vi "Module_IniFile.vi"(7 "処理":enum16{"Read", "Get", "GetArray"}(ring), 8 "error in (no error)":errorcluster caption="エラー入力 (エラーなし)", 9 "一括取得キー":string[](array[string]), 10 "取得キー":string, 11 "ファイルパス":path=path "C:/Users/0128712/Documents/ヘルプファイル/LabVIEW/SampleVI/設定ファイル/ResolverAdj.dat") -> (0 "error out":errorcluster caption="エラー出力", 1 "一括取得データ":string[](array[string]), 3 "取得データ":string)   [LabVIEW 2018]
uses:
  <vilib>/Utility/config.llb/Read Key (String).vi
  <vilib>/Utility/config.llb/NI_LVConfig.lvlib
panel:
  out "読出値":T1(array[cluster])
  # "<機能>\n■Read\n　設定ファイルを読み込む\n　テキスト形式で有れば拡張子は問わない\n■Get\n　キーから値を取得する\n■GetArray\n　キーの配列からまとめて値を取得する\n　Getを複数まとめて行う"
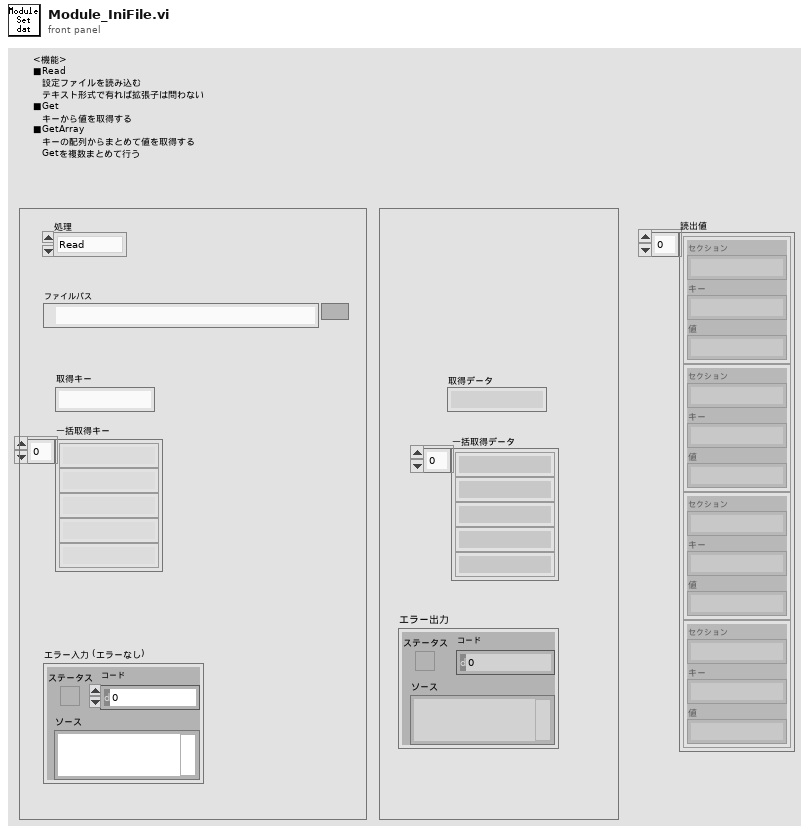
[diagram p1: front panel]
types:
  T1 = cluster{"セクション":string, "キー":string, "値":string}[]
  T2 = typedef "NI_LVConfig.lvlib/Config Data RefNum.ctl" = refnum<k1>
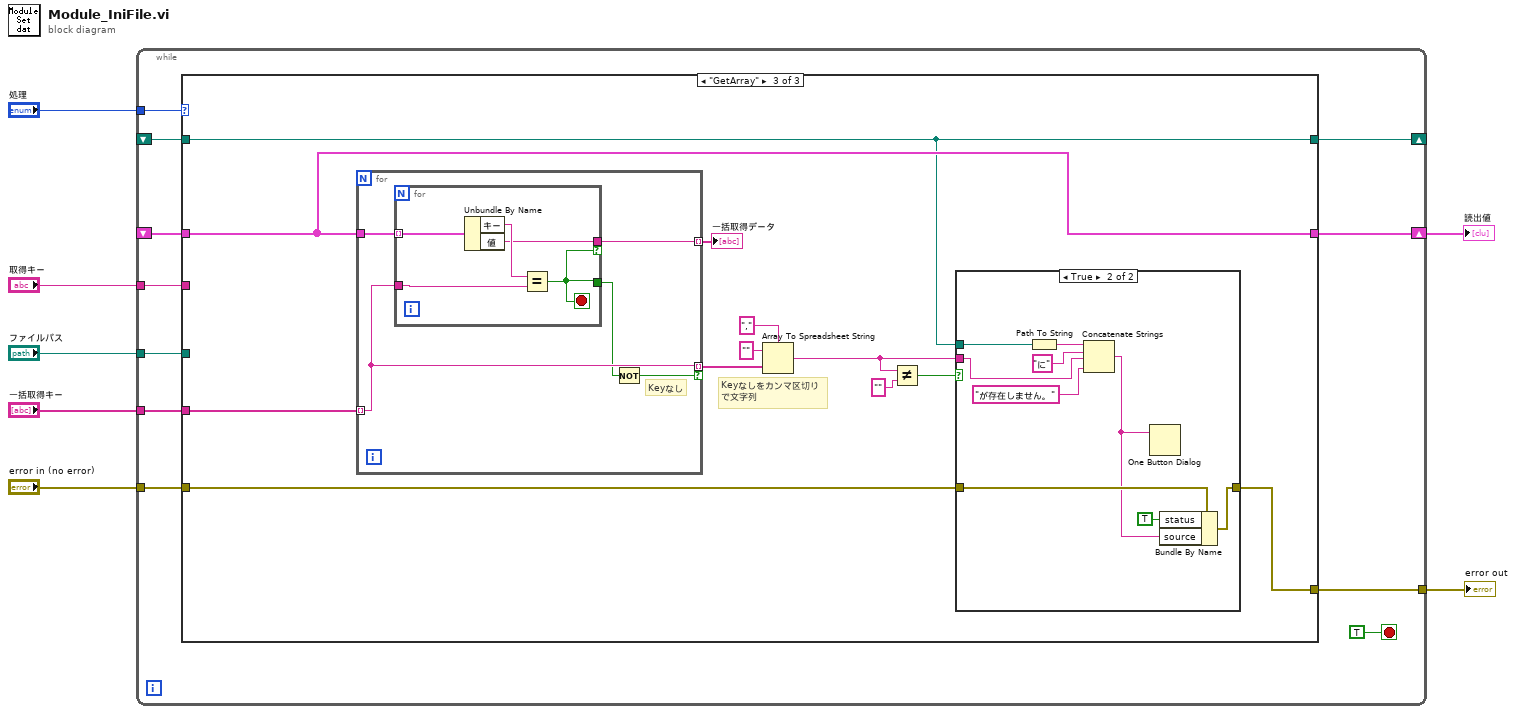
[diagram p0: block diagram]
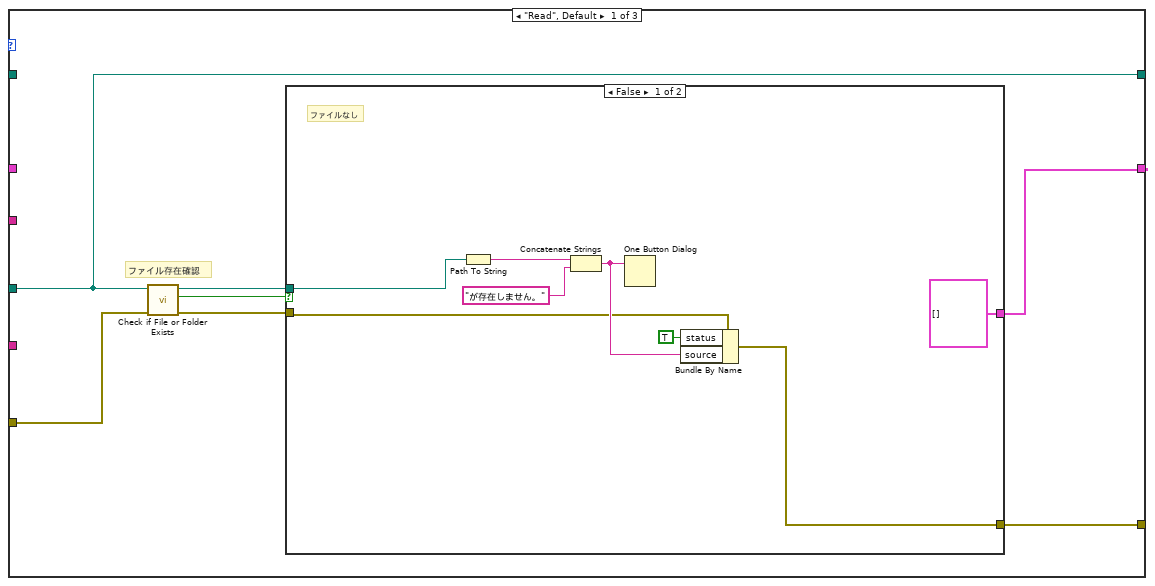
[diagram p2: hidden frame]
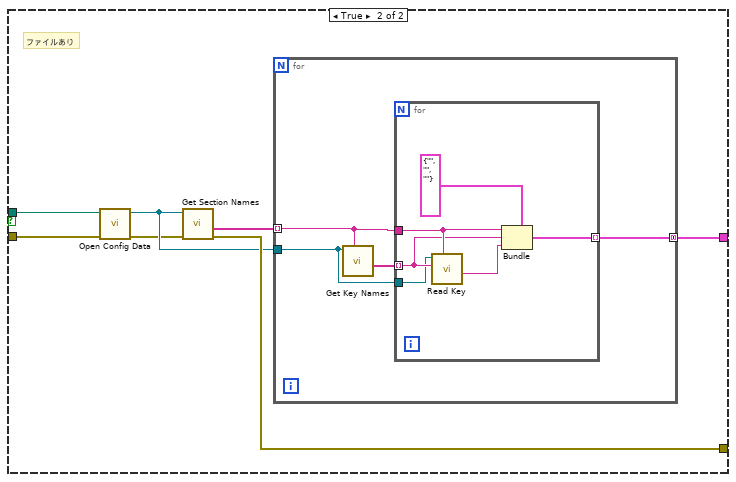
[diagram p3: hidden frame]
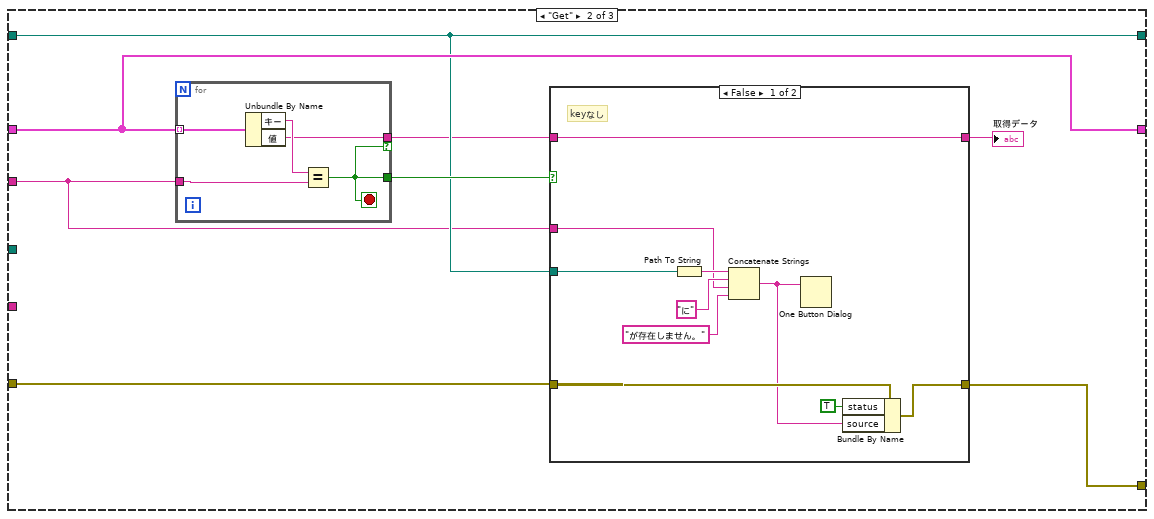
[diagram p4: hidden frame]
diagram:
  n1 = while {
    tunnel: "処理" -> [w17]
    tunnel: "ファイルパス" -> [w16]
    shift-right: [w15] -> w1
    shift-left: _ -> [w14]
    tunnel: "取得キー" -> [w13]
    tunnel: "error in (no error)" -> [w12]
    tunnel: [w11] -> w3
    tunnel: "一括取得キー" -> [w10]
    shift-right: [w9] -> _
    shift-left: _ -> [w8]
    stop <- TRUE stop-if-true
    n2 = case shown="\"GetArray\"" w17 {
      tunnel: w16 -> [w19 _ _]
      tunnel: [w24 w58 w87] -> w15
      tunnel: w14 -> [_ w58 w87]
      tunnel: w13 -> [_ w52 _]
      tunnel: w12 -> [w23 w55 w83]
      tunnel: [w25 w54 w82] -> w11
      tunnel: w10 -> [_ _ w86]
      tunnel: [w19 w53 w84] -> w9
      tunnel: w8 -> [_ w53 w84]
      frame "Read", Default {
        # "ファイル存在確認"
        n3 = call <vilib>:"Check if File or Folder Exists.vi"("error in (no error)"=w23, "path"=w19) -> ("error out"=w22:errorcluster, "file or folder exists?"=w20:bool, "dup path"=w21:path)  [unwired: 7 in]
        n4 = case shown="FALSE" w20 {
          tunnel: [w28 w40] -> w25
          tunnel: [T1 [] w36] -> w24
          tunnel: w22 -> [w29 w35]
          tunnel: w21 -> [w26 w34]
          frame False {
            # "ファイルなし"
            n5 = Path To String(path=w26) -> (string=w33:string)
            n6 = Concatenate Strings(w33, "が存在しません。") -> (w30:string)
            n7 = One Button Dialog(message=w30) -> ()  [unwired: 1 in, 1 out]
            n8 = Bundle By Name(cluster=w29, "status"=TRUE, "source"=w30) -> (w28:errorcluster)
          }
          frame True {
            # "ファイルあり"
            n9 = call <vilib>:"Open Config Data.vi"("error in (no error)"=w35, "configuration file path"=w34) -> ("error out"=w37:errorcluster, "refnum"=w38:T2)  [unwired: 7 in, 1 out]
            n10 = call <vilib>:"Get Section Names.vi"("error in (no error)"=w37, "refnum"=w38) -> ("error out"=w40:errorcluster, "section names"=w39:string[])  [unwired: 7 in, 1 out]
            n11 = for {
              tunnel: w39 -> [w43] mode=indexing
              tunnel: w38 -> [w42]
              tunnel: [w41] -> w36 mode=concatenating
              n12 = call <vilib>:"Get Key Names.vi"("section"=w43, "refnum"=w42) -> ("key names"=w44:string[])  [unwired: 6 in, 3 out]
              n13 = for {
                tunnel: w44 -> [w49] mode=indexing
                tunnel: w43 -> [w50]
                tunnel: w42 -> [w47]
                tunnel: [w46] -> w41 mode=indexing
                n14 = call-poly <vilib>:"Read Key.vi"("section"=w50, "key"=w49, "refnum"=w47) -> ("value"=w48:string)  [unwired: 5 in, 3 out]
                n15 = Bundle(cluster=cluster{"セクション":string, "キー":string, "値":string} {"セクション"="", "キー"="", "値"=""} ("クラスタ 2"), "セクション"=w50, "キー"=w49, "値"=w48) -> (w46:cluster{"セクション":string, "キー":string, "値":string})
              }
            }
          }
        }
      }
      frame "Get" {
        n16 = for {
          tunnel: w58 -> [w75] mode=indexing
          tunnel: w52 -> [w73]
          tunnel: [w72] -> w51 if=w71
          tunnel: [w71] -> w57
          stop <- w71 stop-if-true
          n17 = Unbundle By Name(w75) -> ("キー"=w74:string, "値"=w72:string)
          n18 = Equal?(x=w74, y=w73) -> (x = y?=w71:bool)
        }
        n19 = case shown="FALSE" w57 {
          tunnel: [w59 w69] -> w56
          tunnel: w55 -> [w64 w70]
          tunnel: [w67 w70] -> w54
          tunnel: w53 -> [w66 _]
          tunnel: w52 -> [w61 _]
          tunnel: w51 -> [w59 w69]
          frame False {
            # "keyなし"
            n20 = Path To String(path=w66) -> (string=w65:string)
            n21 = Concatenate Strings(w65, "に", w61, "が存在しません。") -> (w60:string)
            n22 = One Button Dialog(message=w60) -> ()  [unwired: 1 in, 1 out]
            n23 = Bundle By Name(cluster=w64, "status"=TRUE, "source"=w60) -> (w67:errorcluster)
          }
          frame True {
          }
        }
        "取得データ" <- w56
      }
      frame "GetArray" {
        # "Keyなしをカンマ区切り\nで文字列"
        n24 = for {
          tunnel: w87 -> [w102]
          tunnel: w86 -> [w100] mode=indexing
          tunnel: [w101] -> w85 mode=indexing
          tunnel: [w100] -> w81 mode=indexing if=w99
          # "Keyなし"
          n25 = for {
            tunnel: w102 -> [w107] mode=indexing
            tunnel: w100 -> [w105]
            tunnel: [w104] -> w101 if=w103
            tunnel: [w103] -> w98
            stop <- w103 stop-if-true
            n26 = Unbundle By Name(w107) -> ("キー"=w106:string, "値"=w104:string)
            n27 = Equal?(x=w106, y=w105) -> (x = y?=w103:bool)
          }
          n28 = Not(x=w98) -> (.not. x?=w99:bool)
        }
        "一括取得データ" <- w85
        n29 = Array To Spreadsheet String(delimiter (Tab)="," ("デリミタ (タブ)"), array=w81, 3:"" ("形式文字列")) -> (spreadsheet string=w76:string)
        n30 = Not Equal?(x=w76, y="" ("形式文字列")) -> (x != y?=w77:bool)
        n31 = case shown="TRUE" w77 {
          tunnel: w84 -> [_ w92]
          tunnel: w83 -> [w88 w97]
          tunnel: [w88 w96] -> w82
          tunnel: w76 -> [_ w90]
          frame False {
          }
          frame True {
            n32 = Path To String(path=w92) -> (string=w94:string)
            n33 = Concatenate Strings(w94, "に", w90, "が存在しません。") -> (w89:string)
            n34 = One Button Dialog(message=w89) -> ()  [unwired: 1 in, 1 out]
            n35 = Bundle By Name(cluster=w97, "status"=TRUE, "source"=w89) -> (w96:errorcluster)
          }
        }
      }
    }
  }
  "読出値" <- w1
  "error out" <- w3
